vi "XY_UnlockMotors_RT.vi"(10 "ReturnDataStatus":T1) -> (2 "Command":string)   [LabVIEW 2017]
uses:
  sobot structures/ReturnDataStatus.ctl
  sobot structures/SoBot_CommandTypes.ctl
  sobot structures/XY_Commands.ctl
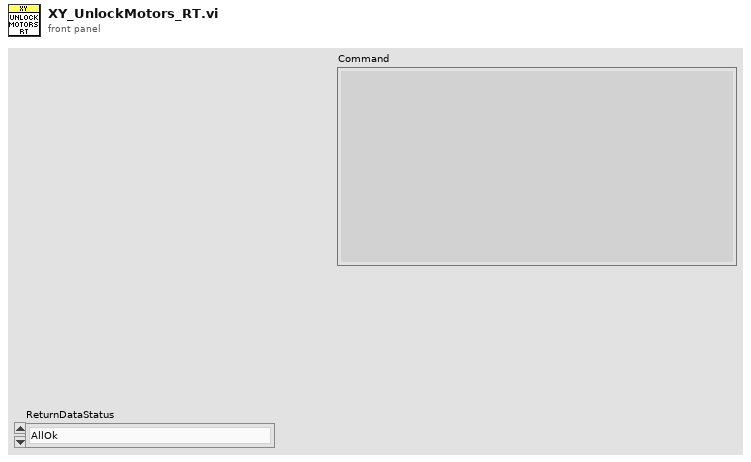
[diagram p1: front panel]
types:
  T1 = typedef "ReturnDataStatus.ctl" = enum16{"AllOk", "Error"}
  T2 = typedef "XY_Commands.ctl" = enum16{"XY_Initialize", "XY_MoveToPosition", "XY_MarkTarget", "XY_LockMotors", "XY_UnlockMotors"}
  T3 = typedef "SoBot_CommandTypes.ctl" = enum16{"General_Command", "XY_Command", "Z_Command", "Plattform_Command"}
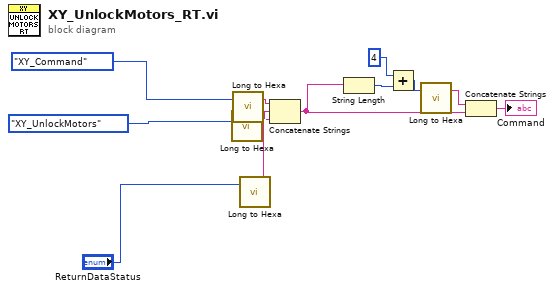
[diagram p0: block diagram]
diagram:
  n1 = call "Long to Hexa.vi"("Long"=XY_Commands."XY_UnlockMotors" ("XY_Command")) -> ("Hexa"=w11:string)  [unwired: 2 in]
  n2 = call "Long to Hexa.vi"("Long"=SoBot_CommandTypes."XY_Command" ("SoBot_CommandTypes")) -> ("Hexa"=w12:string)  [unwired: 2 in]
  n3 = call "Long to Hexa.vi"("Long"="ReturnDataStatus") -> ("Hexa"=w1:string)  [unwired: 2 in]
  n4 = Concatenate Strings(w12, w11, w1) -> (w6:string)
  n5 = String Length(string=w6) -> (length=w10:i32)
  n6 = Add(x=4, y=w10) -> (x+y=w8:i32)
  n7 = call "Long to Hexa.vi"("Long"=w8) -> ("Hexa"=w7:string)  [unwired: 2 in]
  n8 = Concatenate Strings(w7, w6) -> (→"Command":string)
